vi "Getting Started (Loopback Test).vi"() -> ()   [LabVIEW 2017, in "My Network Host v1.lvlib"]
uses:
  My Network Host v1.lvlib
  <vilib>/userdefined/Silver/nirio_resource_slv.ctl
  <instrlib>/_niInstr/FIFO Register Bus/v1/Host/niInstr FIFO Register Bus v1 Host.lvclass
  C:/Program Files (x86)/National Instruments/LabVIEW 2017/instr.lib/_niInstr/Instruction Framework/v1/Host/Instruction Target/niInstr Instruction Target v1 Host.lvclass
  <vilib>/Utility/error.llb/Error Cluster From Error Code.vi
  <vilib>/rvi/errors/niLvFpgaAdjustHostInterfaceError.vi
  <instrlib>/_niInstr/Streaming/v1/Host/Public/Start Finite Stream.vi
  <vilib>/FPGAPlugInAG/Dynamic/niLvFpga_Close_Dynamic.vi
  <vilib>/rvi/interface/nirviReadWriteControl/nirviReadWriteControl.xnode
  <vilib>/rvi/interface/nirviCloseFPGA/nirviCloseFPGA.xnode
  <instrlib>/_niInstr/Instruction Framework/v1/Host/Subsystem Map/niInstr Subsystem Map v1 Host.lvclass
  <instrlib>/_niInstr/Network/API/v1/Host/niInstr Network API Host v1.lvclass
  <instrlib>/_niInstr/Streaming/v1/Host/niInstr Streaming v1 Host.lvlib
  NiFpgaLv.dll
  <vilib>/rvi/interface/Simulation/niFpgaSimulationCallBeginRW.vi
panel:
  in  "RX Instance":i32
  in  "TX Instance":i32=1
  in  "RX IP Address":string="169.254.122.137"
  in  "UDP Destination Port":u16=35311
  out "Data":u8[](array[numeric]) format="%02x"
  out "RX Waveform":u8[](graph)
  out "CLIP state":T1
  out "error out":errorcluster
  in  "resource name":T2="RIO0"
  in  "TX IP Address":string="169.254.122.138"
  # "Example Setup\nNote: Compile the \"TenGbE_Project\" FPGA Target before running this VI. Error 7 \"File not found\" most likely means the bitfile has not been compiled yet.\n\n1. Choose the resource name for your device\n2. Plug a SFP+ Direct Attach cable to the RX Port and to the transmitting Ethernet port\n3. Choose a MAC Source Address for your port.  This needs to be a unique number on the network this is attached to, and is the MAC address for the FPGA network interface\n4. Determine a unique Local IP Address for the FPGA\n5. Run this VI \n6. Run a program capable of sending data to the specified UDP Destination Port/Local IP Address"
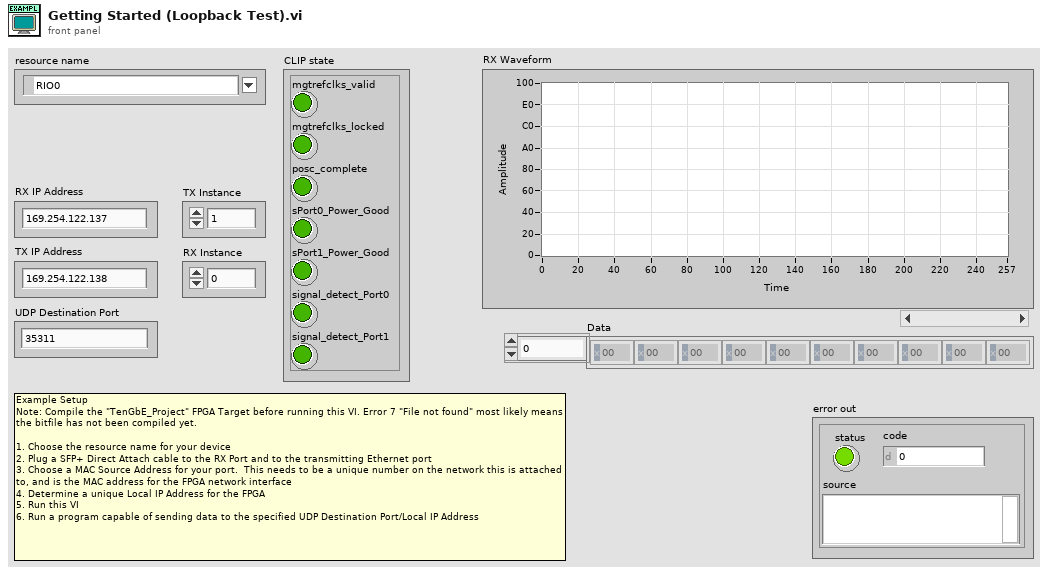
[diagram p1: front panel]
types:
  T1 = cluster{"mgtrefclks_valid":bool, "mgtrefclks_locked":bool, "posc_complete":bool, "sPort0_Power_Good":bool, "sPort1_Power_Good":bool, "signal_detect_Port0":bool, "signal_detect_Port1":bool}
  T2 = typedef "nirio_resource_slv.ctl" = tag
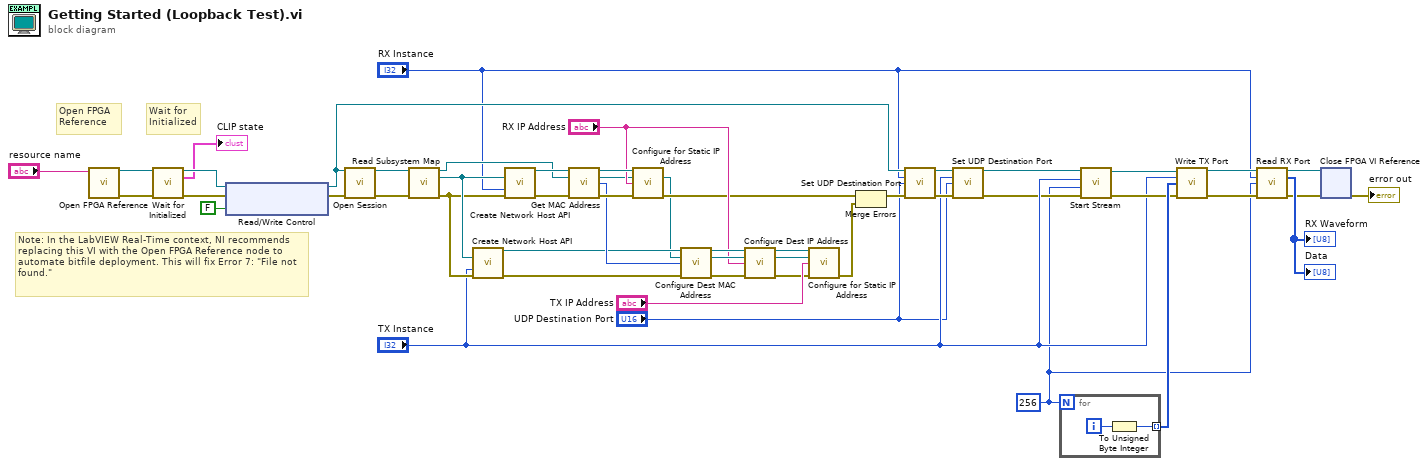
[diagram p0: block diagram]
diagram:
  w4 = 256
  # "Wait for\nInitialized"
  # "Open FPGA\nReference"
  # "Note: In the LabVIEW Real-Time context, NI recommends replacing this VI with the Open FPGA Reference node to automate bitfile deployment. This will fix Error 7: \"File not found.\""
  n1 = call "Open FPGA Reference.vi"("resource name"="resource name") -> ("FPGA VI Reference Out"=w47:refnum<k20>, "error out"=w48:errorcluster)  [unwired: 13 in]
  n2 = call "Wait for Initialized.vi"("Refnum in"=w47, "error in (no error)"=w48) -> ("Refnum out"=w46:refnum<k20>, "CLIP state"=→"CLIP state":T1, "error out"=w40:errorcluster)  [unwired: 11 in]
  n3 = xnode "Read/Write Control"("FPGA VI Reference In"=w46, "error in"=w40, "Use Pattern Gen"=FALSE) -> ("FPGA VI Reference Out"=w42:refnum<k20>, "error out"=w39:errorcluster)
  n4 = call <instrlib>:"Open Session.vi"("fpga ref"=w42, "error in"=w39) -> ("session out"=w51:refnum<class "niInstr FIFO Register Bus v1 Host.lvclass">, "error out"=w50:errorcluster)  [unwired: 12 in]
  n5 = call <instrlib>:"Read Subsystem Map.vi"("instruction target in"=w51, "error in"=w50) -> ("instruction target out"=w23:refnum<class "niInstr FIFO Register Bus v1 Host.lvclass">, "subsystem map"=w31:refnum<class "niInstr Subsystem Map v1 Host.lvclass">, "error out"=w27:errorcluster)  [unwired: 11 in]
  n6 = call <instrlib>:"Create Network Host API.vi"("subsystem map"=w31, "instance number"="TX Instance", "error in (no error)"=w27) -> ("niInstr Network API Host v1 out"=w24:refnum<class "niInstr Network API Host v1.lvclass">, "error out"=w25:errorcluster)  [unwired: 11 in]
  n7 = call <instrlib>:"Create Network Host API.vi"("subsystem map"=w31, "instance number"="RX Instance", "error in (no error)"=w27) -> ("niInstr Network API Host v1 out"=w38:refnum<class "niInstr Network API Host v1.lvclass">, "error out"=w30:errorcluster)  [unwired: 11 in]
  n8 = call <instrlib>:"Get MAC Address.vi"("niInstr Network API Host v1 in"=w38, "instruction target in"=w23, "error in (no error)"=w30) -> ("niInstr Network API Host v1 out"=w37:refnum<class "niInstr Network API Host v1.lvclass">, "instruction target out"=w3:refnum<class "niInstr FIFO Register Bus v1 Host.lvclass">, "Local MAC Address"=w28:u64, "error out"=w36:errorcluster)  [unwired: 9 in]
  n9 = call <instrlib>:"Configure for Static IP Address.vi"("niInstr Network API Host v1 in"=w37, "instruction target in"=w3, "Local IP Address"="RX IP Address", "error in (no error)"=w36) -> ("instruction target out"=w2:refnum<class "niInstr FIFO Register Bus v1 Host.lvclass">, "error out"=w18:errorcluster)  [unwired: 9 in, 1 out]
  n10 = call <instrlib>:"Configure Dest MAC Address.vi"("niInstr Network API Host v1 in"=w24, "instruction target in"=w2, "MAC Destination Address"=w28, "error in (no error)"=w25) -> ("niInstr Network API Host v1 out"=w34:refnum<class "niInstr Network API Host v1.lvclass">, "instruction target out"=w35:refnum<class "niInstr FIFO Register Bus v1 Host.lvclass">, "error out"=w33:errorcluster)  [unwired: 9 in]
  n11 = call <instrlib>:"Configure Dest IP Address.vi"("niInstr Network API Host v1 in"=w34, "instruction target in"=w35, "Dest IP Address"="RX IP Address", "error in (no error)"=w33) -> ("niInstr Network API Host v1 out"=w20:refnum<class "niInstr Network API Host v1.lvclass">, "instruction target out"=w21:refnum<class "niInstr FIFO Register Bus v1 Host.lvclass">, "error out"=w26:errorcluster)  [unwired: 9 in]
  n12 = call <instrlib>:"Configure for Static IP Address.vi"("niInstr Network API Host v1 in"=w20, "instruction target in"=w21, "Local IP Address"="TX IP Address", "error in (no error)"=w26) -> ("error out"=w22:errorcluster)  [unwired: 9 in, 2 out]
  n13 = Merge Errors(w18, w22) -> (w19:errorcluster)
  n14 = call "Set UDP Destination Port.vi"("Refnum in"=w42, "ethernet port"="RX Instance", "UDP Destination Port"="UDP Destination Port", "error in (no error)"=w19) -> ("Refnum out"=w10:refnum<k20>, "error out"=w9:errorcluster)  [unwired: 10 in]
  n15 = call "Set UDP Destination Port.vi"("Refnum in"=w10, "ethernet port"="TX Instance", "UDP Destination Port"="UDP Destination Port", "error in (no error)"=w9) -> ("Refnum out"=w5:refnum<k20>, "error out"=w6:errorcluster)  [unwired: 10 in]
  n16 = for {
    N: w4 -> [_]
    tunnel: [w52] -> w17 mode=indexing
    i -> [w53]
    n17 = To Unsigned Byte Integer(number=w53) -> (unsigned 8bit integer=w52:u8)
  }
  n18 = call-poly <instrlib>:"Start Stream.vi"("error in (no error)"=w6, "num samples"=w4, "stream index"="TX Instance", "refnum in"=w5) -> ("error out"=w16:errorcluster, "refnum out"=w15:refnum<k20>)  [unwired: 6 in]
  n19 = call "Write TX Port.vi"("Refnum in"=w15, "TX Port"="TX Instance", "Data"=w17, "error in (no error)"=w16) -> ("Refnum out"=w12:refnum<k20>, "error out"=w13:errorcluster)  [unwired: 10 in]
  n20 = call "Read RX Port.vi"("Refnum in"=w12, "Ethernet port"="RX Instance", "Elements to Read"=w4, "error in (no error)"=w13) -> ("Refnum out"=w43:refnum<k20>, "Data"=→"Data" →"RX Waveform":u8[], "error out"=w11:errorcluster)  [unwired: 8 in, 1 out]
  n21 = xnode "Close FPGA VI Reference"("FPGA VI Reference In"=w43, "error in"=w11) -> ("error out"=→"error out":errorcluster)
